vi "Write Channel scanner configuration.vi"(8 "error in (no error)":errorcluster, 10 "Configuration":T1, 11 "Channel Scanner in":refnum<class "Channel Scanner.lvclass">) -> (0 "error out":errorcluster, 3 "Channel Scanner out":refnum<class "Channel Scanner.lvclass">)   [LabVIEW 2016, in "Channel Scanner.lvclass"]
uses:
  Channel Scanner.lvclass
  C:/github/Measure_core/da Base/Template Module.lvclass
  Channel Scanner Configuration.ctl
  Measure_core/Template Module/Template Module.lvclass/Template Module.ctl
  Measure_core/Template Module/Write Configuration.vi
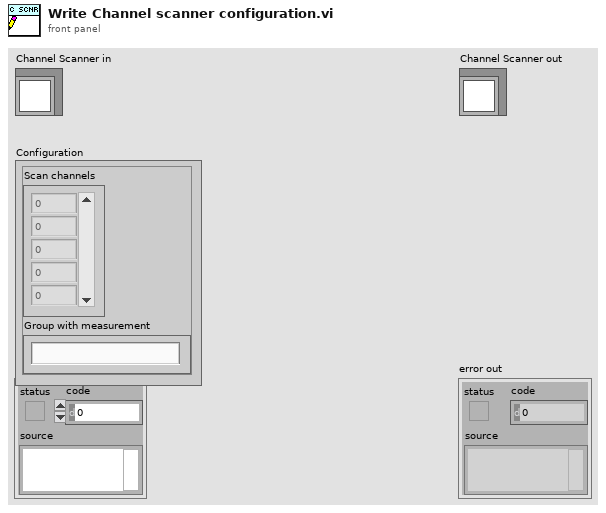
[diagram p1: front panel]
types:
  T1 = typedef "Channel Scanner Configuration.ctl" = cluster{"Scan channels":i32[], "Group with measurement":string}
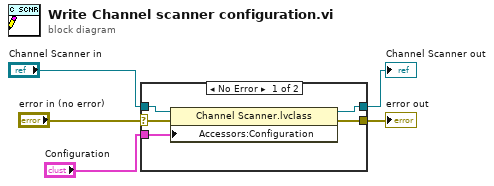
[diagram p0: block diagram]
diagram:
  n1 = case shown="No Error" "error in (no error)" {
    selector: "error in (no error)" -> [w7 w11]
    tunnel: [w6 w11] -> w4
    tunnel: [w9 w12] -> w2
    tunnel: "Channel Scanner in" -> [w10 w12]
    tunnel: "Configuration" -> [w8 _]
    frame No Error {
      n2 = property class="Channel Scanner.lvclass"(reference=w10, error in=w7, "Accessors:Configuration"=w8) -> (reference out=w9:refnum<class "Channel Scanner.lvclass">, error out=w6:errorcluster)
    }
    frame Error {
    }
  }
  "error out" <- w4
  "Channel Scanner out" <- w2
